vi "Read Attribute Notes.vi"(11 "Sequence Dialog in":refnum<class "Sequence Dialog.lvclass">) -> (2 "Attribute Notes":string[](array[string]), 3 "Sequence Dialog out":refnum<class "Sequence Dialog.lvclass">)   [LabVIEW 2017, in "Sequence Dialog.lvclass"]
uses:
  <vilib>/gpm_packages/@cs/Test-executive-builder/Source/Test Executive Builder Dialogs/Edit Sequence Dialog/Sequence Dialog.lvclass
  <vilib>/gpm_packages/@cs/Test-executive-builder/Source/Test Executive Builder Dialogs/Edit Sequence Dialog/Sequence Dialog.lvclass/Sequence Dialog.ctl
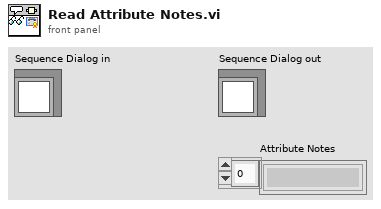
[diagram p1: front panel]
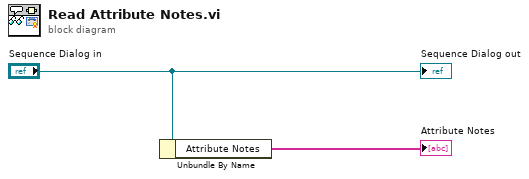
[diagram p0: block diagram]
diagram:
  n1 = Unbundle By Name("Sequence Dialog in") -> ("Attribute Notes"=→"Attribute Notes":string[])
  "Sequence Dialog out" <- "Sequence Dialog in"
